vi "manifold config to odor set (sub-vi).vi"(10 "manifold configuration":T1) -> (2 "utilized odor set":set{T6}(c389))   [LabVIEW 2021]
uses:
  type-defs/odor selection (type def).ctl
  type-defs/manifold configuration cluster array (type def).ctl
  type-defs/manifold configuration cluster (type def).ctl
  type-defs/manifold selection.ctl
  type-defs/single port single odor cluster.ctl
  type-defs/port number (type def).ctl
  type-defs/odor color (type def).ctl
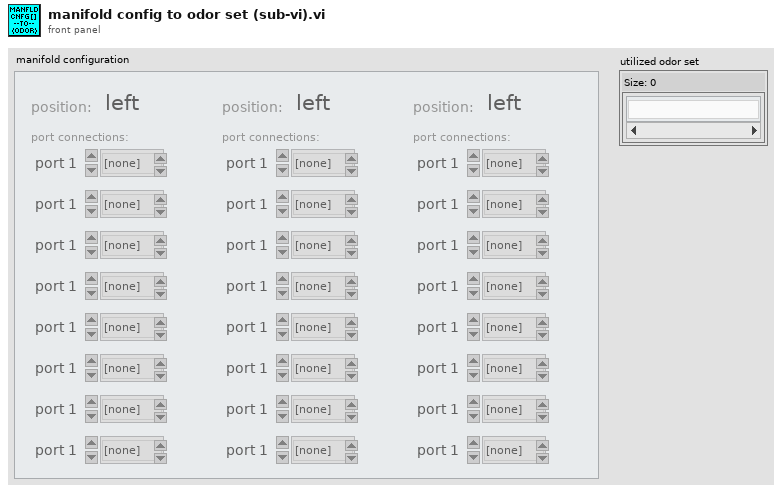
[diagram p1: front panel]
types:
  T1 = typedef "manifold configuration cluster array (type def).ctl" = T2[]
  T2 = typedef "manifold configuration cluster (type def).ctl" = cluster{"position:":T3, "port connections:":T4[]}
  T3 = typedef "manifold selection.ctl" = enum16{"left", "middle", "right"}
  T4 = typedef "single port single odor cluster.ctl" = cluster{"port number":T5, "connected odor":T6, "error":bool, "odor color":T7}
  T5 = typedef "port number (type def).ctl" = enum16{"port 1", "port 2", "port 3", "port 4", "port 5", "port 6", "port 7", "port 8"}
  T6 = typedef "odor selection (type def).ctl" = enum16{"[none]", "odor 1", "odor 2", "odor 3", "odor 4", "odor 5", "odor 6", "odor 7", "odor 8", "odor 9", "odor 10"}
  T7 = typedef "odor color (type def).ctl" = u16
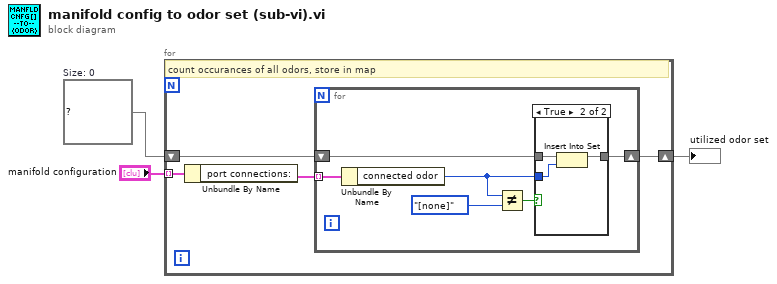
[diagram p0: block diagram]
diagram:
  w3 = set{T6} {}  # Size: 0
  n1 = for {
    shift-right: [w5] -> w2
    shift-left: w3 -> [w6]
    tunnel: "manifold configuration" -> [w4] mode=indexing
    # "count occurances of all odors, store in map"
    n2 = Unbundle By Name(w4) -> ("port connections:"=w7:T4[])
    n3 = for {
      tunnel: w7 -> [w13] mode=indexing
      shift-right: [w12] -> w5
      shift-left: w6 -> [w11]
      n4 = Unbundle By Name(w13) -> ("connected odor"=w10:T6)
      n5 = Not Equal?(x=w10, y=odor_selection_(type_def)."[none]" ("connected odor")) -> (x != y?=w8:bool)
      n6 = case shown="True" w8 {
        tunnel: [w14 w16] -> w12
        tunnel: w11 -> [w14 w17]
        tunnel: w10 -> [_ w15]
        frame False {
        }
        frame True {
          n7 = Insert Into Set(10:w15, 11:w17) -> (3:w16:set{T6})  [unwired: 1 out]
        }
      }
    }
  }
  "utilized odor set" <- w2
